vi "ReadCompiled.vi"(0 "Compiled String":string="#DopplerCooling\r\n0.9 10100000 00000000 00000000\r\n\r\n#Pump\r\n0.3 01000000 00000000 00000000\r\n\r\n#Pulsed\r\n0.2 00100000 00000000 00000000\r\n0.4 00000100 00000000 00000000\r\n0.2 00000000 10000000 00000000\r\n0.2 01000000 00000000 01000000\n") -> (1 "Durations":dbl[](array[numeric]), 2 "States":string[](array[string]), 3 "ChapterNames":string[](array[string]), 4 "ChapterPositions":u32[](array[numeric]))   [LabVIEW 2011]
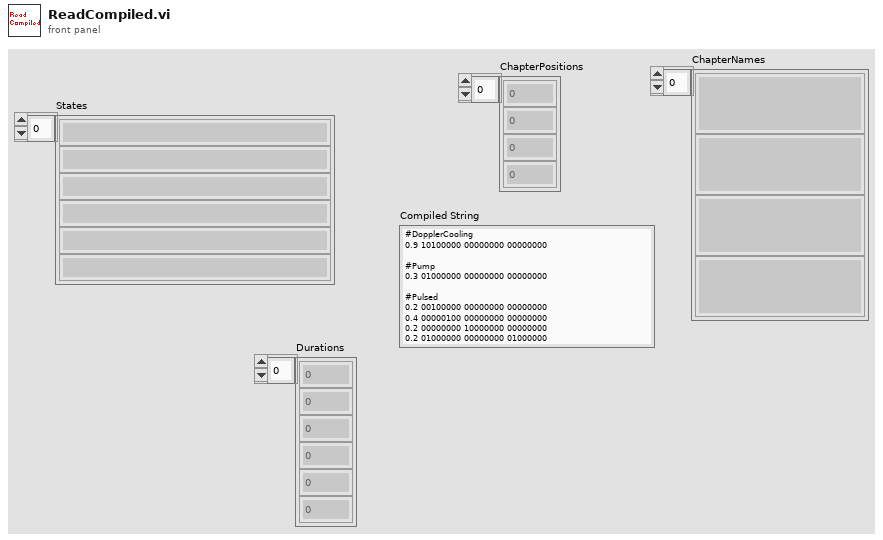
[diagram p1: front panel]
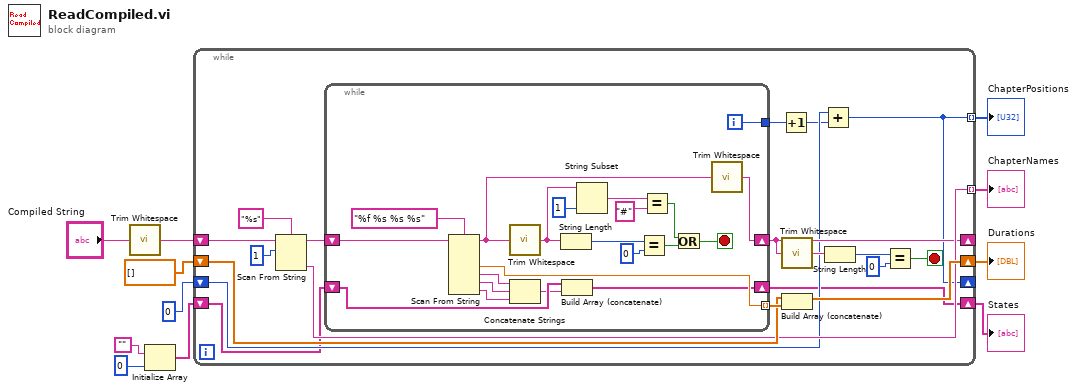
[diagram p0: block diagram]
diagram:
  n1 = call <vilib>:"Trim Whitespace.vi"("string"="Compiled String") -> ("trimmed string"=w1:string)  [unwired: 1 in]
  n2 = Initialize Array("", 0 ("dimension size")) -> (w6:string[])
  n3 = while {
    shift-right: [w27] -> w11
    shift-left: dbl[] [] -> [w25]
    tunnel: [w24] -> w9 mode=indexing
    shift-right: [w19] -> _
    shift-left: w1 -> [w23]
    shift-right: [w14] -> _
    shift-left: u32 0 ("initial scan location") -> [w16]
    tunnel: [w14] -> w7 mode=indexing
    shift-right: [w12] -> w3
    shift-left: w6 -> [w13]
    stop <- w20 stop-if-true
    n4 = Scan From String(format string="%s", input string=w23, initial scan location=u32 1) -> (remaining string=w29:string, output 1=w24:string)  [unwired: 2 in, 2 out]
    n5 = while {
      tunnel: [w49] -> w26 mode=indexing
      shift-right: [w43] -> w19
      shift-left: w29 -> [w51]
      tunnel: [w34] -> w17
      shift-right: [w31] -> w12
      shift-left: w13 -> [w33]
      i -> [w34]
      stop <- w37 stop-if-true
      n6 = Scan From String(format string="%f %s %s %s", input string=w51) -> (remaining string=w36:string, output 1=w49:dbl, output 2=w48:string, output 3=w47:string, output 4=w46:string)  [unwired: 6 in, 2 out]
      n7 = call <vilib>:"Trim Whitespace.vi"("string"=w36) -> ("trimmed string"=w35:string)  [unwired: 1 in]
      n8 = Concatenate Strings(w48, w47, w46) -> (w32:string)
      n9 = String Length(string=w35) -> (length=w45:i32)
      n10 = Build Array (concatenate)(w33, w32) -> (w31:string[])
      n11 = String Subset(string=w35, length (rest)=1 ("line index")) -> (substring=w41:string)  [unwired: 1 in]
      n12 = Equal?(x=w45, y=0) -> (x = y?=w38:bool)
      n13 = Equal?(x=w41, y="#") -> (x = y?=w39:bool)
      n14 = Or(x=w39, y=w38) -> (x .or. y?=w37:bool)
      n15 = call <vilib>:"Trim Whitespace.vi"("string"=w36) -> ("trimmed string"=w43:string)  [unwired: 1 in]
    }
    n16 = Increment(x=w17) -> (x+1=w15:i32)
    n17 = call <vilib>:"Trim Whitespace.vi"("string"=w19) -> ("trimmed string"=w18:string)  [unwired: 1 in]
    n18 = Build Array (concatenate)(w25, w26) -> (w27:dbl[])
    n19 = Add(x=w16, y=w15) -> (x+y=w14:u32)
    n20 = String Length(string=w18) -> (length=w22:i32)
    n21 = Equal?(x=w22, y=0) -> (x = y?=w20:bool)
  }
  "Durations" <- w11
  "ChapterNames" <- w9
  "ChapterPositions" <- w7
  "States" <- w3
